vi "PalmSense Configure CV.vi"(8 "error in (no error)":errorcluster, 10 "Message Data":variant, 11 "Data Cluster in":T1) -> (0 "error out":errorcluster, 3 "Data Cluster out":T1)   [LabVIEW 2020, in "PalmSens.lvlib"]
uses:
  PalmSens.lvlib
  PalmSense Hardware Configuration.ctl
  <instrlib>/PalmSens SDK for LabVIEW 5.10/PalmSens/PalmSens.lvclass
  support/Message Queue/Message Cluster.ctl
  support/HW Message Cluster.ctl
  C:/Program Files (x86)/National Instruments/LabVIEW 2020/instr.lib/PalmSens SDK for LabVIEW 5.10/PalmSens/Libraries/PalmSens.Core.dll
  support/Message Queue/Message Queue.lvlib
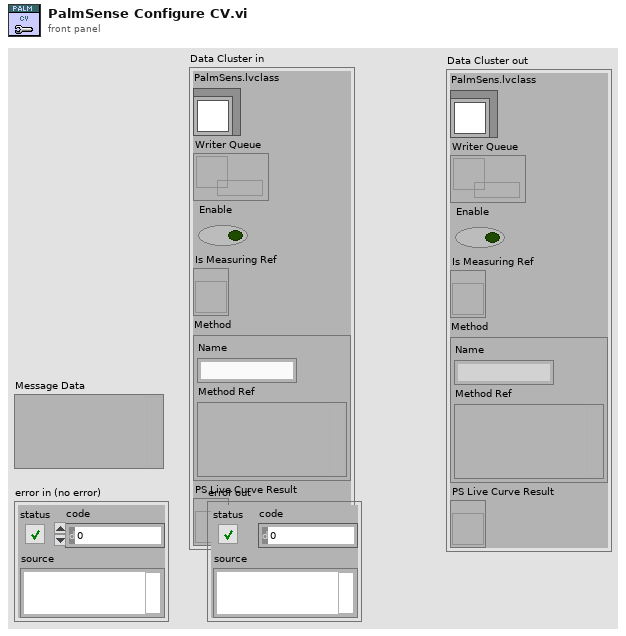
[diagram p1: front panel]
types:
  T1 = typedef "PalmSens.lvlib/PalmSense Hardware Configuration.ctl" = cluster{"PalmSens.lvclass":refnum<class "PalmSens.lvclass">, "Writer Queue":refnum<queue>, "Enable":bool, "Is Measuring Ref":refnum<vi>, "Method":cluster{"Name":string, "Method Ref":variant}, "PS Live Curve Result":refnum<vi>}
  T2 = cluster{"BeginPotential":dbl, "Vtx1Potential":dbl, "Vtx2Potential":dbl, "StepPotential":dbl, "Scanrate":dbl, "nScans":dbl}
  T3 = typedef "Message Queue.lvlib/HW Message Cluster.ctl" = cluster{"Writer Queue":refnum<queue>, "Writer Data":T4}
  T4 = typedef "Message Queue.lvlib/Message Cluster.ctl" = cluster{"Message":string, "Message Data":variant}
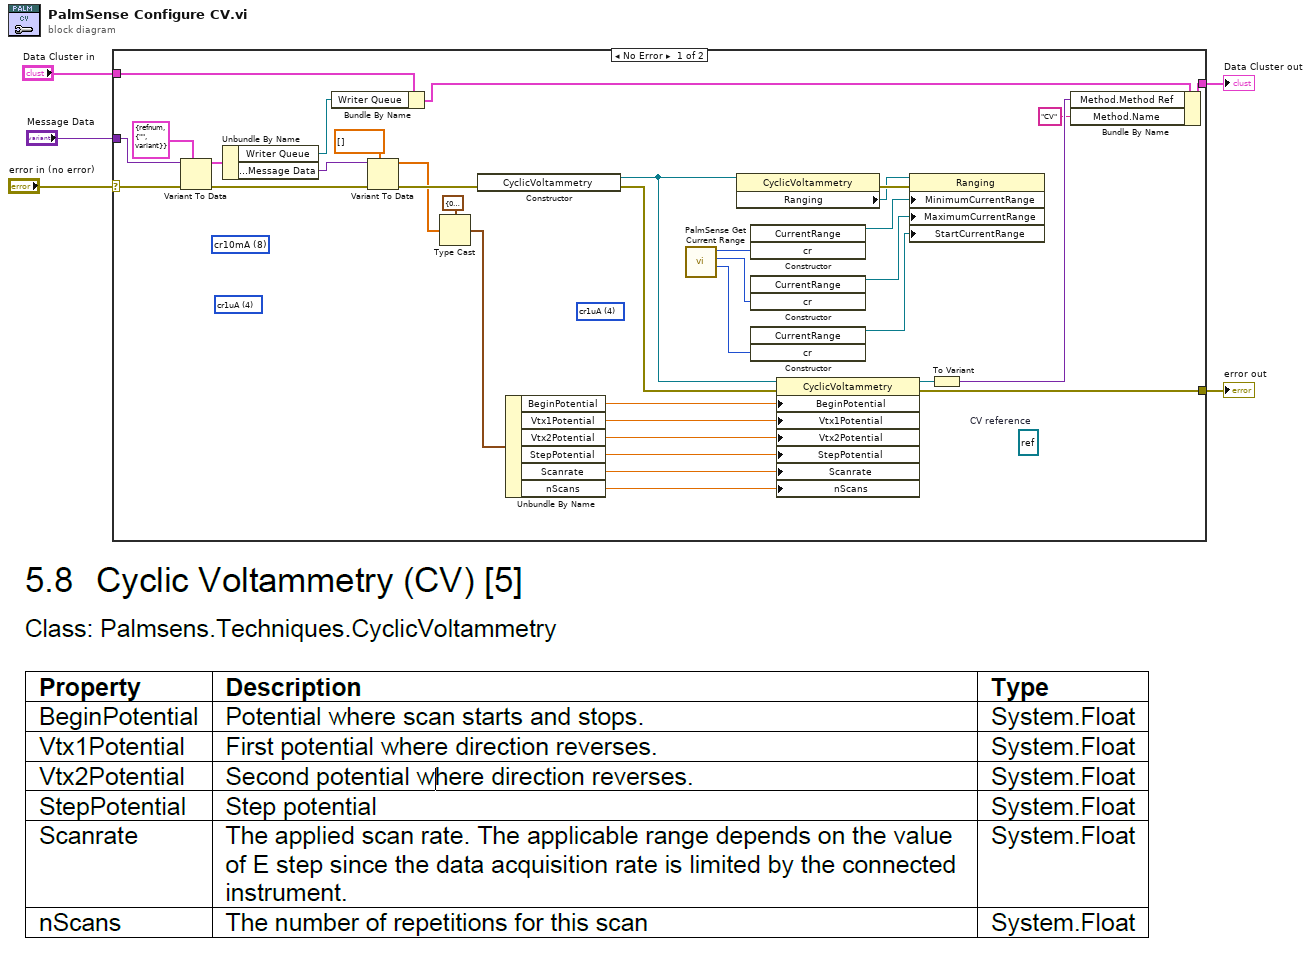
[diagram p0: block diagram]
diagram:
  n1 = case shown="No Error" "error in (no error)" {
    selector: "error in (no error)" -> [w37 w41]
    tunnel: "Message Data" -> [w35 _]
    tunnel: [w16 w42] -> w4
    tunnel: "Data Cluster in" -> [w39 w42]
    tunnel: [w20 w41] -> w2
    frame No Error {
      (unwired) 4 items=["cr100pA"=0, "cr1nA"=1, "cr10nA"=2, "cr100nA"=3, "cr1uA"=4, "cr10uA"=5, "cr100uA"=6, "cr1mA"=7, "cr10mA"=8, "cr100mA"=9, "cr2uA"=10, "cr4uA"=11, "cr8uA"=12, "cr16uA"=13, "cr32uA"=14, "cr125uA"=17, "cr250uA"=18, "cr500uA"=19, "cr5mA"=20, "cr6uA"=21, "cr13uA"=22, "cr25uA"=23, "cr50uA"=24, "cr200uA"=25, "cr63uA"=26] ("cr")
      (unwired) 4 items=["cr100pA"=0, "cr1nA"=1, "cr10nA"=2, "cr100nA"=3, "cr1uA"=4, "cr10uA"=5, "cr100uA"=6, "cr1mA"=7, "cr10mA"=8, "cr100mA"=9, "cr2uA"=10, "cr4uA"=11, "cr8uA"=12, "cr16uA"=13, "cr32uA"=14, "cr125uA"=17, "cr250uA"=18, "cr500uA"=19, "cr5mA"=20, "cr6uA"=21, "cr13uA"=22, "cr25uA"=23, "cr50uA"=24, "cr200uA"=25, "cr63uA"=26] ("cr")
      (unwired) 8 items=["cr100pA"=0, "cr1nA"=1, "cr10nA"=2, "cr100nA"=3, "cr1uA"=4, "cr10uA"=5, "cr100uA"=6, "cr1mA"=7, "cr10mA"=8, "cr100mA"=9, "cr2uA"=10, "cr4uA"=11, "cr8uA"=12, "cr16uA"=13, "cr32uA"=14, "cr125uA"=17, "cr250uA"=18, "cr500uA"=19, "cr5mA"=20, "cr6uA"=21, "cr13uA"=22, "cr25uA"=23, "cr50uA"=24, "cr200uA"=25, "cr63uA"=26] ("cr")
      (unwired) refnum<k24> refnum  # CV reference
      n2 = Variant To Data(error in=w37, type=T3 {"Writer Queue"=refnum, "Writer Data"={"Message"="", "Message Data"=variant}}, Variant=w35) -> (data=w38:T3, error out=w36:errorcluster)
      n3 = Unbundle By Name(w38) -> ("Writer Queue"=w33:refnum<queue>, "Writer Data.Message Data"=w34:variant)
      n4 = Bundle By Name(cluster=w39, "Writer Queue"=w33) -> (w40:T1)
      n5 = Variant To Data(error in=w36, type=dbl[] [] ("LSV Scan"), Variant=w34) -> (data=w11:dbl[], error out=w31:errorcluster)
      n6 = Type Cast(type=T2 {"BeginPotential"=0.0, "Vtx1Potential"=0.0, "Vtx2Potential"=0.0, "StepPotential"=0.0, "Scanrate"=0.0, "nScans"=0.0} ("cluster"), x=w11) -> (*(type *) &x=w9:T2)
      n7 = constructor class="CyclicVoltammetry"(error in=w31) -> (reference out=w29:refnum<k24>, error out=w30:errorcluster)  [unwired: 2 in, 1 out]
      n8 = Unbundle By Name(w9) -> ("BeginPotential"=w26:dbl, "Vtx1Potential"=w25:dbl, "Vtx2Potential"=w24:dbl, "StepPotential"=w23:dbl, "Scanrate"=w22:dbl, "nScans"=w21:dbl)
      n9 = call "PalmSense Get Current Range.vi"() -> ("Start Current Range"=w6:i32, "Max Current Range"=w7:i32, "Min Current Range"=w8:i32)  [unwired: 9 in]
      n10 = property class="CyclicVoltammetry"(reference=w29) -> (error out=w28:errorcluster, "Ranging"=w27:refnum<k24>)  [unwired: 1 in, 1 out]
      n11 = constructor class="CurrentRange"("cr"=w8) -> (reference out=w19:refnum<k24>)  [unwired: 3 in, 3 out]
      n12 = constructor class="CurrentRange"("cr"=w7) -> (reference out=w18:refnum<k24>)  [unwired: 3 in, 3 out]
      n13 = constructor class="CurrentRange"("cr"=w6) -> (reference out=w17:refnum<k24>)  [unwired: 3 in, 3 out]
      n14 = property class="CyclicVoltammetry"(reference=w29, error in=w30, "BeginPotential"=w26, "Vtx1Potential"=w25, "Vtx2Potential"=w24, "StepPotential"=w23, "Scanrate"=w22, "nScans"=w21) -> (reference out=w15:refnum<k24>, error out=w20:errorcluster)
      n15 = property class="Ranging"(reference=w27, error in=w28, "MinimumCurrentRange"=w19, "MaximumCurrentRange"=w18, "StartCurrentRange"=w17) -> ()  [unwired: 2 out]
      n16 = To Variant(anything=w15) -> (Variant=w14:variant)
      n17 = Bundle By Name(cluster=w40, "Method.Method Ref"=w14, "Method.Name"="CV") -> (w16:T1)
    }
    frame Error {
    }
  }
  "Data Cluster out" <- w4
  "error out" <- w2
